vi "corrector.vi"(10 "Array":dbl[](array[numeric])) -> (2 "valor salida":dbl)   [LabVIEW 2018]
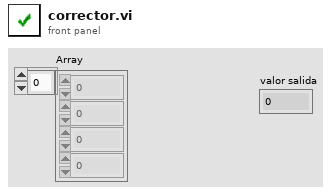
[diagram p1: front panel]
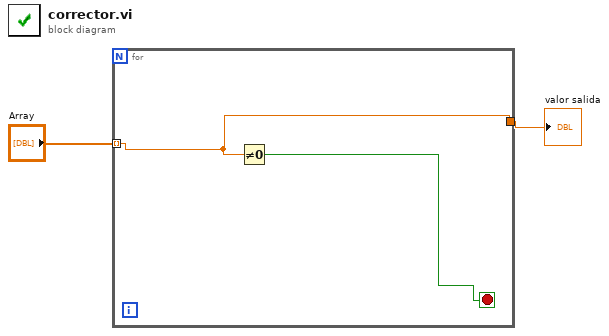
[diagram p0: block diagram]
diagram:
  n1 = for {
    tunnel: "Array" -> [w3] mode=indexing
    tunnel: [w3] -> w1
    stop <- w4 stop-if-true
    n2 = Not Equal To 0?(x=w3) -> (x != 0?=w4:bool)
  }
  "valor salida" <- w1
